vi "Debouncer_Reset.vi"(8 "CurrentTIme":dbl=-1.0, 11 "Debouncer In":T1 {"PrevTimeSeconds" format="%13.6p"; "DebounceTimeSeconds" format="%13.6p"}) -> (0 "CurrentTIme Out":dbl=-1.0, 3 "Debouncer Out":T1 {"PrevTimeSeconds" format="%13.6p"; "DebounceTimeSeconds" format="%13.6p"})   [LabVIEW 2019, in "Trajectory_Library.lvlib"]
doc: "This is an internal function.\n\nResets previous time."
uses:
  Trajectory_Library.lvlib
  TypeDef/DEBOUNCER.ctl
  Enum/DEBOUNCER_TYPE_ENUM.ctl
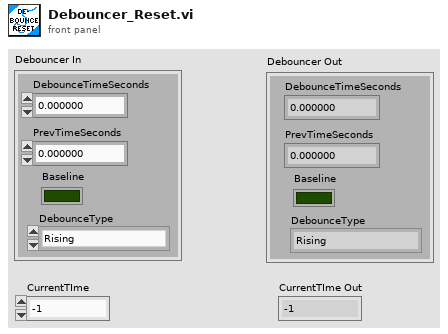
[diagram p1: front panel]
types:
  T1 = typedef "Trajectory_Library.lvlib/DEBOUNCER.ctl" = cluster{"DebounceTimeSeconds":dbl, "PrevTimeSeconds":dbl, "Baseline":bool, "DebounceType":T2}
  T2 = typedef "Trajectory_Library.lvlib/DEBOUNCER_TYPE_ENUM.ctl" = enum16{"Rising", "Falling", "Both"}
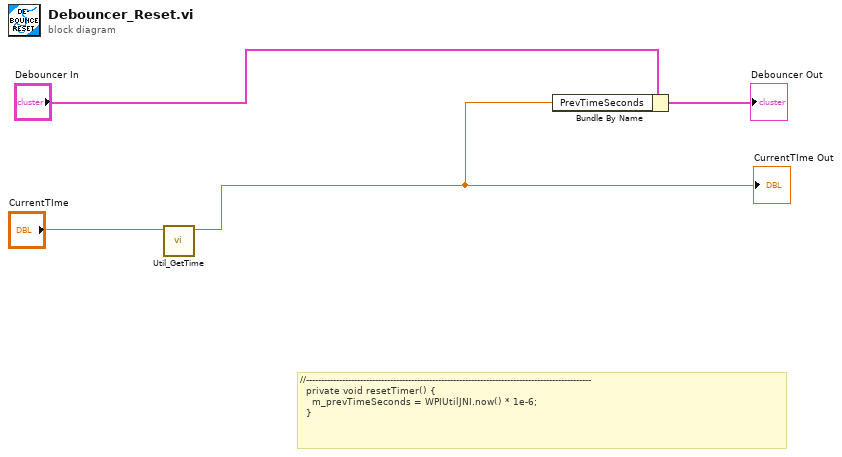
[diagram p0: block diagram]
diagram:
  # "//-----------------------------------------------------------------------------------------------\n  private void resetTimer() {\n    m_prevTimeSeconds = WPIUtilJNI.now() * 1e-6;\n  }"
  n1 = call "Util_GetTime.vi"("Pass_Through_Time"="CurrentTIme") -> ("FPGA_Time_Seconds"=w2:dbl)  [unwired: 8 in, 2 out]
  "CurrentTIme Out" <- w2
  n2 = Bundle By Name(cluster="Debouncer In", "PrevTimeSeconds"=w2) -> (→"Debouncer Out":T1)
